vi "标样核查.vi"() -> ()   [LabVIEW 2016, in "斯坦道多参数.lvlib"]
panel:
  out "运行状态":u16(ring) items=["空闲", "水样测试", "标样核查"]
  out "seconds since 1Jan1904":timestamp
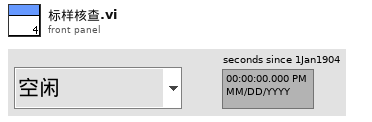
[diagram p1: front panel]
types:
  T1 = cluster{"ph":bool, "DO":bool, "Cond":bool, "Turb":bool, "叶绿素a":bool, "藻密度":bool, "ORP":bool, "cod":bool, "DO2":bool, "氯化物":bool, "氨氮":bool, "水中油":bool, "悬浮物":bool, "余氯":bool}
  T2 = cluster{"运行模式":enum16{"维护模式", "常规模式", "应急模式", "质控模式"}, "24H周期设置":bool[]}
  T3 = typedef "集成多参数单参数字段定义.ctl" = cluster{"时间":timestamp, "测量模式":string, "数据类型":string, "检测值":sgl, "单位":string, "数据标识":string, "信号值":sgl, "标样参考值":sgl, "因子编码":string, "探头温度":sgl, "LastTime":timestamp}
  T4 = cluster{"数据保存间隔":dbl, "保存组数":dbl, "水温标样值":dbl, "pH标样值":dbl, "溶解氧标样值":dbl, "电导率标样值":dbl, "浊度标样值":dbl, "悬浮物标样值":dbl, "叶绿素a标样值":dbl, "藻密度标样值":dbl, "ORP标样值":dbl, "氯化物标样值":dbl, "COD标样值":dbl, "氨氮标样值":dbl, "水中油标样值":dbl, "余氯标样值":dbl, "pH启用":bool, "溶解氧启用":bool, "电导率启用":bool, "浊度启用":bool, "悬浮物启用":bool, "叶绿素a启用":bool, "藻密度启用":bool, "ORP启用":bool, "氯化物启用":bool, "COD启用":bool, "氨氮启用":bool, "水中油启用":bool, "余氯启用":bool}
  T5 = typedef "LVDateTimeRec.ctl" = cluster{"秒数的小数部分":dbl, "秒":i32, "分":i32, "时":i32, "日":i32, "月":i32, "年":i32, "天数（周）":i32, "天数（年）":i32, "DST":i32}
  T6 = cluster{"温度测量值":sgl, "测量值":sgl, "温度偏移修正值":sgl, "信号值":sgl, "数据标识":string}
  T7 = cluster{"温度测量值":sgl, "DO%":sgl, "DOmg/L":sgl, "温度偏移修正值":sgl, "数据标识mg/L":string, "数据标识%":string}
  T8 = cluster{"CH":u16, "监测值":dbl, "信号值":sgl, "数据标识":string}
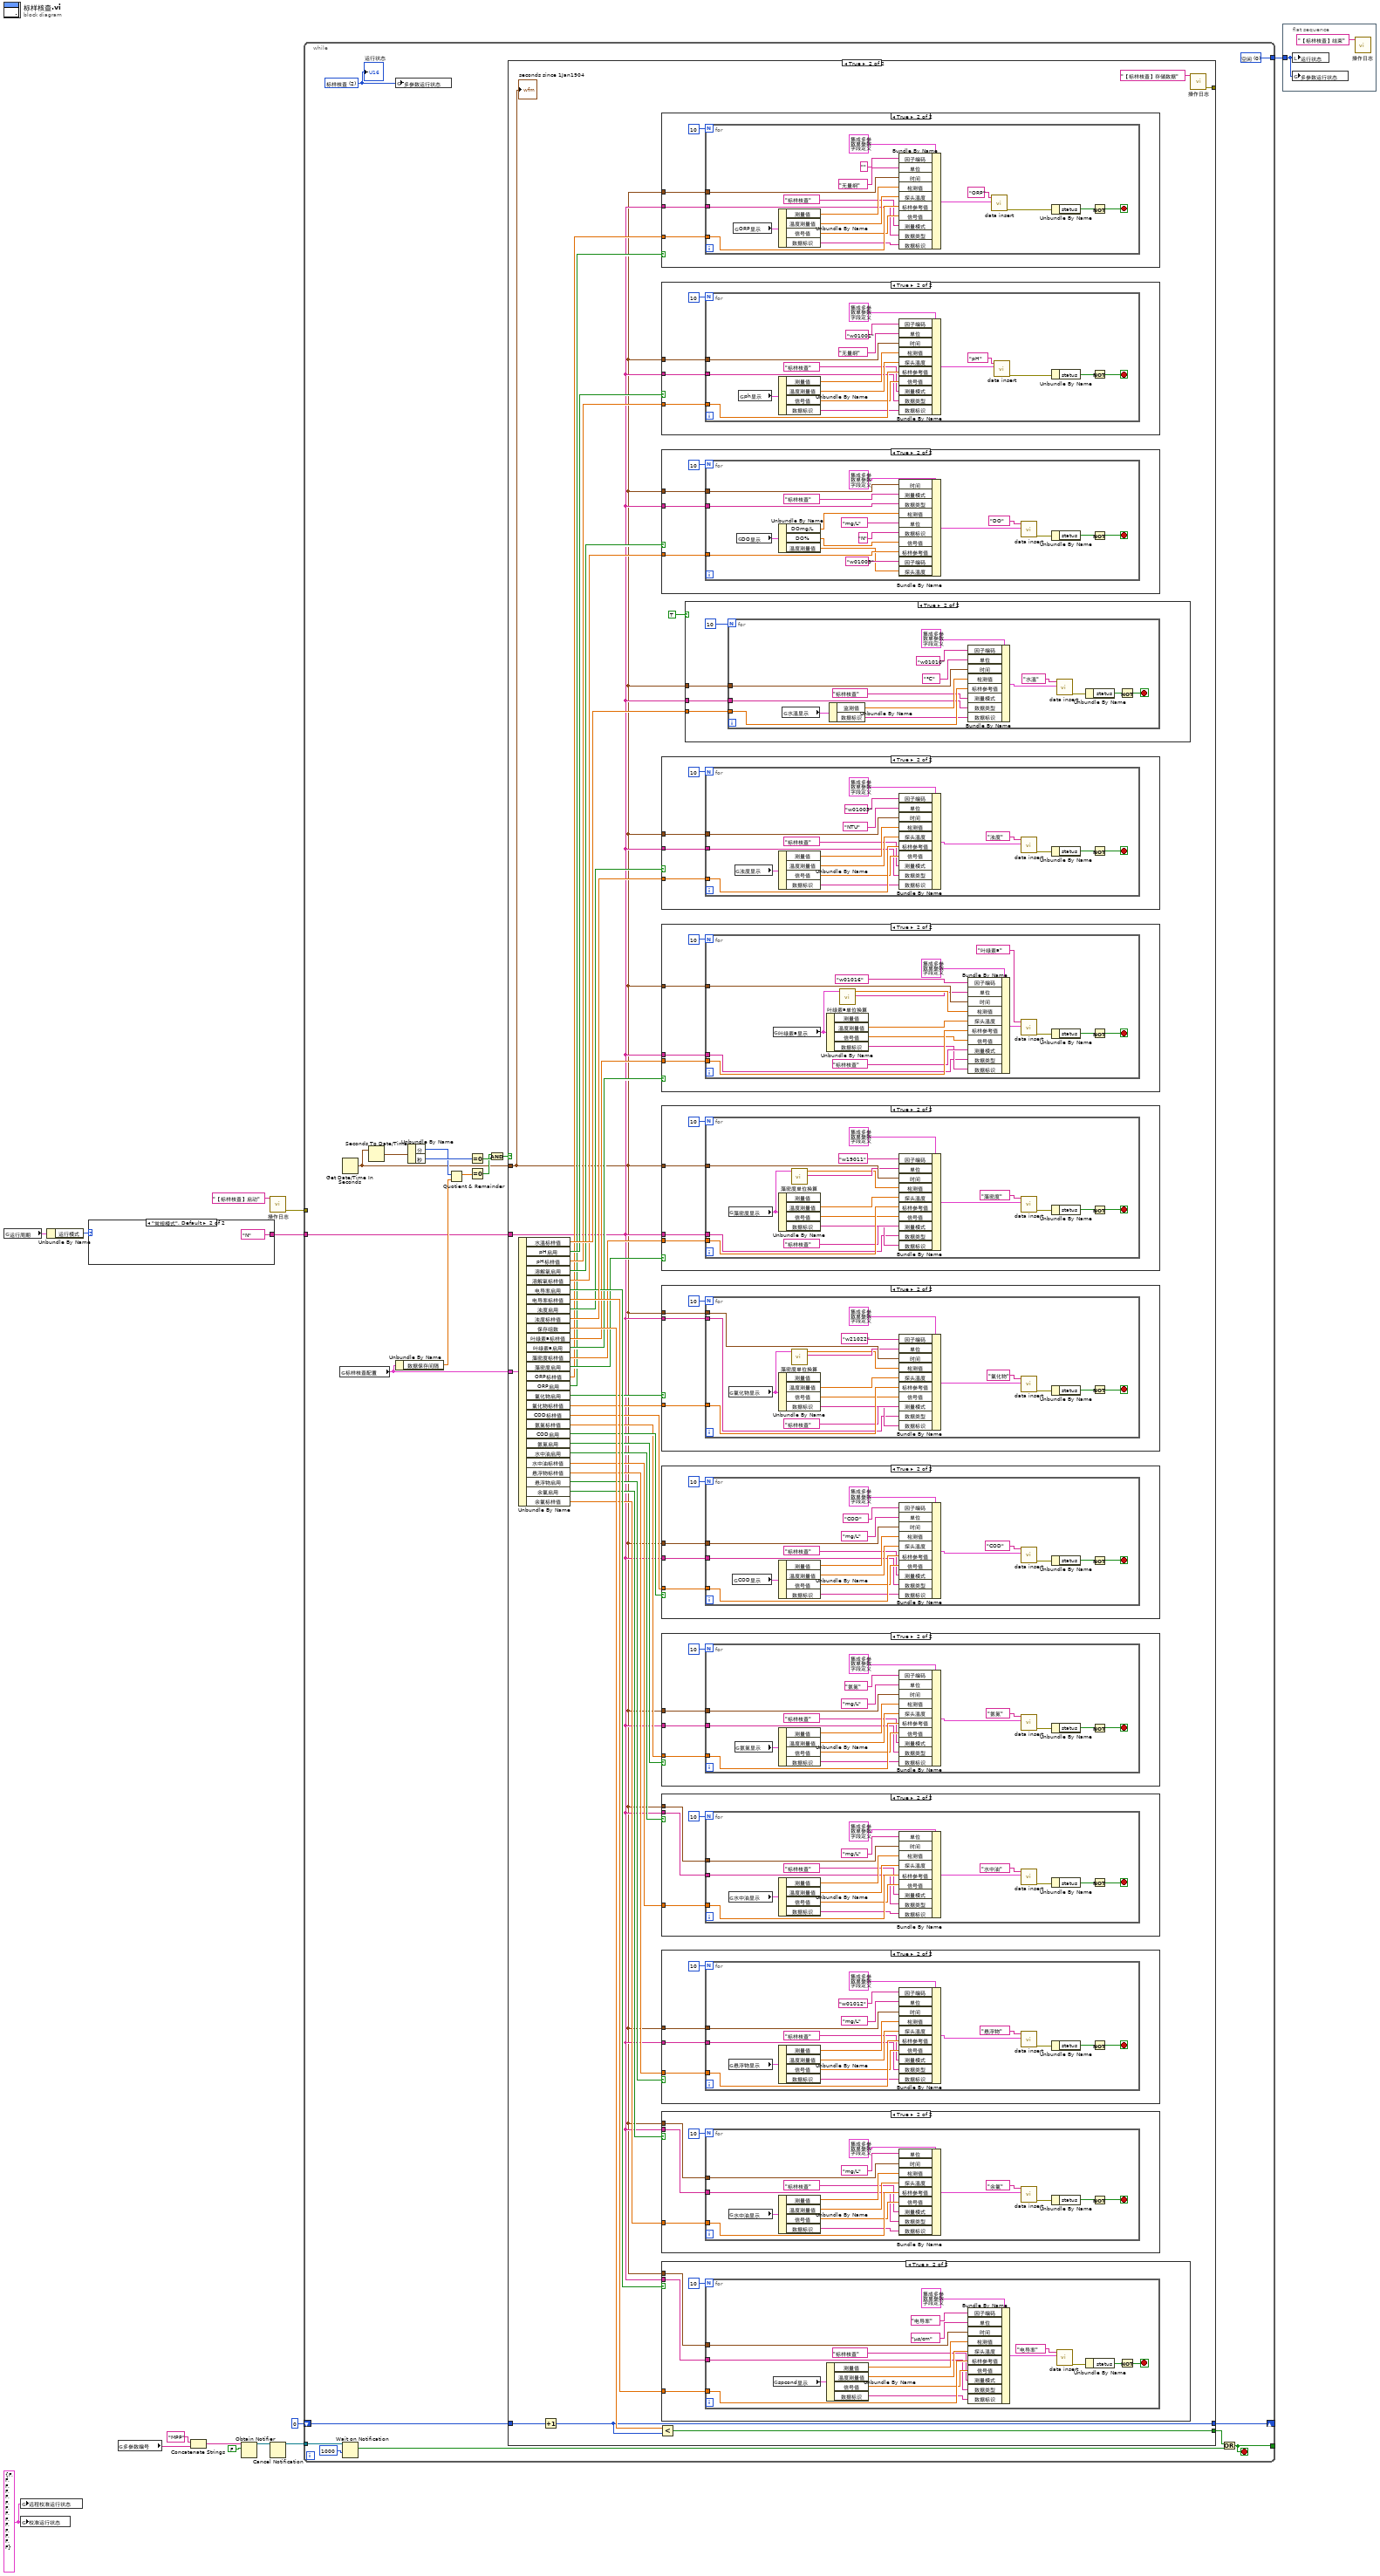
[diagram p0: block diagram]
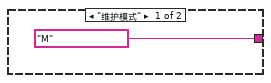
[diagram p2: hidden frame]
diagram:
  w1 = T1 {"ph"=FALSE, "DO"=FALSE, "Cond"=FALSE, "Turb"=FALSE, "叶绿素a"=FALSE, "藻密度"=FALSE, "ORP"=FALSE, "cod"=FALSE, "DO2"=FALSE, "氯化物"=FALSE, "氨氮"=FALSE, "水中油"=FALSE, "悬浮物"=FALSE, "余氯"=FALSE} ("远程校准运行状态")
  n1 = global read "断电保存变量.vi" "运行周期"() -> (w3:T2)
  n2 = global write "多参数全局变量.vi" "远程校准运行状态"(w1) -> ()
  n3 = global write "多参数全局变量.vi" "校准运行状态"(w1) -> ()
  n4 = Unbundle By Name(w3) -> ("运行模式"=w2:enum16{"维护模式", "常规模式", "应急模式", "质控模式"})
  n5 = case shown="\"常规模式\", Default" w2 {
    tunnel: ["M" ("数据标记表") "N" ("数据标记表")] -> w4
    frame "维护模式" {
    }
    frame "常规模式", Default {
    }
  }
  n6 = global read "多参数全局变量.vi" "多参数编号"() -> (w8:string)
  n7 = Concatenate Strings("MPP" ("名称（未命名）"), w8) -> (w9:string)
  n8 = Obtain Notifier(name (unnamed)=w9, notification data type=FALSE) -> (notifier out=w12:refnum<notifier>)  [unwired: 2 in, 2 out]
  n9 = call "操作日志.vi"("日志信息"="【标样核查】启动") -> ("error out"=w6:errorcluster)  [unwired: 10 in]
  n10 = Cancel Notification(0:w12) -> (8:w11:refnum<notifier>)  [unwired: 1 in, 2 out]
  n11 = while {
    tunnel: [w27] -> w10
    tunnel: w11 -> [w26]
    tunnel: w6 -> [_]
    shift-right: [w20] -> _
    shift-left: 0 -> [w21]
    tunnel: w4 -> [w18]
    tunnel: [w17] -> _
    stop <- w17 stop-if-true
    w27 = u16 0 items=["空闲", "水样测试", "标样核查"] ("多参数运行状态")
    w23 = u16 2 items=["空闲", "水样测试", "标样核查"] ("多参数运行状态")
    n12 = global read "断电保存变量.vi" "标样核查配置"() -> (w22:T4)
    n13 = Get Date/Time In Seconds() -> (seconds since 1Jan1904=w28:timestamp)
    n14 = Wait on Notification(notifier=w26, timeout in ms (-1)=1000 ("超时毫秒(-1)")) -> (notification=w24:bool)  [unwired: 2 in, 3 out]
    n15 = Seconds To Date/Time(time stamp (now)=w28) -> (date time rec=w36:T5)  [unwired: 1 in]
    n16 = global write "多参数全局变量.vi" "多参数运行状态"(w23) -> ()
    n17 = Unbundle By Name(w22) -> ("数据保存间隔"=w31:dbl)
    n18 = Unbundle By Name(w36) -> ("分"=w32:i32, "秒"=w35:i32)
    n19 = Quotient & Remainder(x=w32, y=w31) -> (x-y*floor(x/y)=w30:dbl)  [unwired: 1 out]
    n20 = Equal To 0?(x=w35) -> (x = 0?=w34:bool)
    n21 = Equal To 0?(x=w30) -> (x = 0?=w29:bool)
    n22 = And(x=w29, y=w34) -> (x .and. y?=w33:bool)
    n23 = case shown="True" w33 {
      tunnel: w22 -> [_ w74]
      tunnel: w28 -> [_ w38]
      tunnel: [_ w67] -> _
      tunnel: w21 -> [w37 w61]
      tunnel: [w37 w59] -> w20
      tunnel: [_ w58] -> w19
      tunnel: w18 -> [_ w39]
      frame False {
      }
      frame True {
        n24 = Unbundle By Name(w74) -> ("水温标样值"=w73:dbl, "pH启用"=w66:bool, "pH标样值"=w72:dbl, "溶解氧启用"=w64:bool, "溶解氧标样值"=w71:dbl, "电导率启用"=w63:bool, "电导率标样值"=w70:dbl, "浊度启用"=w62:bool, "浊度标样值"=w69:dbl, "保存组数"=w60:dbl, "叶绿素a标样值"=w57:dbl, "叶绿素a启用"=w54:bool, "藻密度标样值"=w56:dbl, "藻密度启用"=w55:bool, "ORP标样值"=w53:dbl, "ORP启用"=w52:bool, "氯化物启用"=w51:bool, "氯化物标样值"=w50:dbl, "COD标样值"=w48:dbl, "氨氮标样值"=w46:dbl, "COD启用"=w49:bool, "氨氮启用"=w47:bool, "水中油启用"=w44:bool, "水中油标样值"=w45:dbl, "悬浮物标样值"=w42:dbl, "悬浮物启用"=w43:bool, "余氯启用"=w41:bool, "余氯标样值"=w40:dbl)
        n25 = Increment(x=w61) -> (x+1=w59:i32)
        n26 = Less?(x=w60, y=w59) -> (x < y?=w58:bool)
        n27 = case shown="True" w52 {
          tunnel: w53 -> [_ w202]
          tunnel: w38 -> [_ w200]
          tunnel: w39 -> [_ w199]
          frame False {
          }
          frame True {
            n28 = for {
              N: 10 -> [_]
              tunnel: w202 -> [w218]
              tunnel: w200 -> [w211]
              tunnel: w199 -> [w206]
              stop <- w212 stop-if-true
              n29 = global read "多参数全局变量.vi" "ORP显示"() -> (w217:T6)
              n30 = Unbundle By Name(w217) -> ("测量值"=w216:sgl, "温度测量值"=w215:sgl, "信号值"=w209:sgl, "数据标识"=w207:string)
              n31 = Bundle By Name(cluster=T3 {"时间"=timestamp(0 s since 1904-01-01), "测量模式"="水样测试", "数据类型"="N", "检测值"=0.0, "单位"="mg/L", "数据标识"="N", "信号值"=0.0, "标样参考值"=0.0, "因子编码"="", "探头温度"=0.0, "LastTime"=timestamp(0 s since 1904-01-01)} ("data"), "因子编码"="", "单位"="无量纲", "时间"=w211, "检测值"=w216, "探头温度"=w215, "标样参考值"=w218, "信号值"=w209, "测量模式"="标样核查", "数据类型"=w206, "数据标识"=w207) -> (w210:T3)
              n32 = call "data insert.vi"("data"=w210, "table in"="ORP") -> ("error out"=w214:errorcluster)  [unwired: 9 in]
              n33 = Unbundle By Name(w214) -> ("status"=w213:bool)
              n34 = Not(x=w213) -> (.not. x?=w212:bool)
            }
          }
        }
        n35 = case shown="True" w66 {
          tunnel: w72 -> [_ w328]
          tunnel: w38 -> [_ w326]
          tunnel: w39 -> [_ w325]
          frame False {
          }
          frame True {
            n36 = for {
              N: 10 -> [_]
              tunnel: w328 -> [w342]
              tunnel: w326 -> [w335]
              tunnel: w325 -> [w330]
              stop <- w336 stop-if-true
              n37 = global read "多参数全局变量.vi" "ph显示"() -> (w341:T6)
              n38 = Unbundle By Name(w341) -> ("测量值"=w340:sgl, "温度测量值"=w339:sgl, "信号值"=w333:sgl, "数据标识"=w331:string)
              n39 = Bundle By Name(cluster=T3 {"时间"=timestamp(0 s since 1904-01-01), "测量模式"="水样测试", "数据类型"="N", "检测值"=0.0, "单位"="mg/L", "数据标识"="N", "信号值"=0.0, "标样参考值"=0.0, "因子编码"="", "探头温度"=0.0, "LastTime"=timestamp(0 s since 1904-01-01)} ("data"), "因子编码"="w01001", "单位"="无量纲", "时间"=w335, "检测值"=w340, "探头温度"=w339, "标样参考值"=w342, "信号值"=w333, "测量模式"="标样核查", "数据类型"=w330, "数据标识"=w331) -> (w334:T3)
              n40 = call "data insert.vi"("data"=w334, "table in"="pH" ("table输入")) -> ("error out"=w338:errorcluster)  [unwired: 9 in]
              n41 = Unbundle By Name(w338) -> ("status"=w337:bool)
              n42 = Not(x=w337) -> (.not. x?=w336:bool)
            }
          }
        }
        n43 = case shown="True" w64 {
          tunnel: w71 -> [_ w307]
          tunnel: w38 -> [_ w305]
          tunnel: w39 -> [_ w304]
          frame False {
          }
          frame True {
            n44 = for {
              N: 10 -> [_]
              tunnel: w307 -> [w314]
              tunnel: w305 -> [w319]
              tunnel: w304 -> [w309]
              stop <- w322 stop-if-true
              n45 = global read "多参数全局变量.vi" "DO显示"() -> (w324:T7)
              n46 = Unbundle By Name(w324) -> ("DOmg/L"=w317:sgl, "DO%"=w311:sgl, "温度测量值"=w310:sgl)
              n47 = Bundle By Name(cluster=T3 {"时间"=timestamp(0 s since 1904-01-01), "测量模式"="水样测试", "数据类型"="N", "检测值"=0.0, "单位"="mg/L", "数据标识"="N", "信号值"=0.0, "标样参考值"=0.0, "因子编码"="", "探头温度"=0.0, "LastTime"=timestamp(0 s since 1904-01-01)} ("data"), "时间"=w319, "测量模式"="标样核查", "数据类型"=w309, "检测值"=w317, "单位"="mg/L", "数据标识"="N" ("水样数据标识"), "信号值"=w311, "标样参考值"=w314, "因子编码"="w01009", "探头温度"=w310) -> (w320:T3)
              n48 = call "data insert.vi"("data"=w320, "table in"="DO") -> ("error out"=w312:errorcluster)  [unwired: 9 in]
              n49 = Unbundle By Name(w312) -> ("status"=w323:bool)
              n50 = Not(x=w323) -> (.not. x?=w322:bool)
            }
          }
        }
        n51 = case shown="True" w62 {
          tunnel: w69 -> [_ w265]
          tunnel: w38 -> [_ w263]
          tunnel: w39 -> [_ w262]
          frame False {
          }
          frame True {
            n52 = for {
              N: 10 -> [_]
              tunnel: w265 -> [w278]
              tunnel: w263 -> [w271]
              tunnel: w262 -> [w267]
              stop <- w272 stop-if-true
              n53 = global read "多参数全局变量.vi" "浊度显示"() -> (w277:T6)
              n54 = Unbundle By Name(w277) -> ("测量值"=w276:sgl, "温度测量值"=w275:sgl, "信号值"=w270:sgl, "数据标识"=w268:string)
              n55 = Bundle By Name(cluster=T3 {"时间"=timestamp(0 s since 1904-01-01), "测量模式"="水样测试", "数据类型"="N", "检测值"=0.0, "单位"="mg/L", "数据标识"="N", "信号值"=0.0, "标样参考值"=0.0, "因子编码"="", "探头温度"=0.0, "LastTime"=timestamp(0 s since 1904-01-01)} ("data"), "因子编码"="w01003", "单位"="NTU", "时间"=w271, "检测值"=w276, "探头温度"=w275, "标样参考值"=w278, "信号值"=w270, "测量模式"="标样核查", "数据类型"=w267, "数据标识"=w268) -> (w281:T3)
              n56 = call "data insert.vi"("data"=w281, "table in"="浊度" ("table输入")) -> ("error out"=w274:errorcluster)  [unwired: 9 in]
              n57 = Unbundle By Name(w274) -> ("status"=w273:bool)
              n58 = Not(x=w273) -> (.not. x?=w272:bool)
            }
          }
        }
        n59 = case shown="True" w54 {
          tunnel: w57 -> [_ w244]
          tunnel: w38 -> [_ w242]
          tunnel: w39 -> [_ w241]
          frame False {
          }
          frame True {
            n60 = for {
              N: 10 -> [_]
              tunnel: w244 -> [w258]
              tunnel: w242 -> [w253]
              tunnel: w241 -> [w249]
              stop <- w254 stop-if-true
              n61 = global read "多参数全局变量.vi" "叶绿素a显示"() -> (w247:T6)
              n62 = Unbundle By Name(w247) -> ("温度测量值"=w257:sgl, "信号值"=w252:sgl, "数据标识"=w250:string)  [unwired: 1 out]
              n63 = call "叶绿素a单位换算.vi"("叶绿素a显示"=w247) -> ("检测值1.单位"=w245:string, "测量值"=w246:sgl)  [unwired: 8 in, 1 out]
              n64 = Bundle By Name(cluster=T3 {"时间"=timestamp(0 s since 1904-01-01), "测量模式"="水样测试", "数据类型"="N", "检测值"=0.0, "单位"="mg/L", "数据标识"="N", "信号值"=0.0, "标样参考值"=0.0, "因子编码"="", "探头温度"=0.0, "LastTime"=timestamp(0 s since 1904-01-01)} ("data"), "因子编码"="w01016", "单位"=w245, "时间"=w253, "检测值"=w246, "探头温度"=w257, "标样参考值"=w258, "信号值"=w252, "测量模式"="标样核查", "数据类型"=w249, "数据标识"=w250) -> (w261:T3)
              n65 = call "data insert.vi"("data"=w261, "table in"="叶绿素a" ("table输入")) -> ("error out"=w256:errorcluster)  [unwired: 9 in]
              n66 = Unbundle By Name(w256) -> ("status"=w255:bool)
              n67 = Not(x=w255) -> (.not. x?=w254:bool)
            }
          }
        }
        n68 = case shown="True" w55 {
          tunnel: w56 -> [_ w223]
          tunnel: w38 -> [_ w221]
          tunnel: w39 -> [_ w220]
          frame False {
          }
          frame True {
            n69 = for {
              N: 10 -> [_]
              tunnel: w223 -> [w237]
              tunnel: w221 -> [w232]
              tunnel: w220 -> [w228]
              stop <- w233 stop-if-true
              n70 = global read "多参数全局变量.vi" "藻密度显示"() -> (w226:T6)
              n71 = Unbundle By Name(w226) -> ("温度测量值"=w236:sgl, "信号值"=w231:sgl, "数据标识"=w229:string)  [unwired: 1 out]
              n72 = call "藻密度单位换算.vi"("藻密度显示"=w226) -> ("检测值1.单位"=w225:string, "测量值"=w224:sgl)  [unwired: 8 in, 1 out]
              n73 = Bundle By Name(cluster=T3 {"时间"=timestamp(0 s since 1904-01-01), "测量模式"="水样测试", "数据类型"="N", "检测值"=0.0, "单位"="mg/L", "数据标识"="N", "信号值"=0.0, "标样参考值"=0.0, "因子编码"="", "探头温度"=0.0, "LastTime"=timestamp(0 s since 1904-01-01)} ("data"), "因子编码"="w19011", "单位"=w225, "时间"=w232, "检测值"=w224, "探头温度"=w236, "标样参考值"=w237, "信号值"=w231, "测量模式"="标样核查", "数据类型"=w228, "数据标识"=w229) -> (w240:T3)
              n74 = call "data insert.vi"("data"=w240, "table in"="藻密度" ("table输入")) -> ("error out"=w235:errorcluster)  [unwired: 9 in]
              n75 = Unbundle By Name(w235) -> ("status"=w234:bool)
              n76 = Not(x=w234) -> (.not. x?=w233:bool)
            }
          }
        }
        n77 = case shown="True" w51 {
          tunnel: w50 -> [_ w181]
          tunnel: w38 -> [_ w179]
          tunnel: w39 -> [_ w178]
          frame False {
          }
          frame True {
            n78 = for {
              N: 10 -> [_]
              tunnel: w181 -> [w197]
              tunnel: w179 -> [w192]
              tunnel: w178 -> [w188]
              stop <- w193 stop-if-true
              n79 = global read "多参数全局变量.vi" "氯化物显示"() -> (w186:T6)
              n80 = Unbundle By Name(w186) -> ("温度测量值"=w196:sgl, "信号值"=w191:sgl, "数据标识"=w189:string)  [unwired: 1 out]
              n81 = call "藻密度单位换算.vi"("藻密度显示"=w186) -> ("检测值1.单位"=w185:string, "测量值"=w184:sgl)  [unwired: 8 in, 1 out]
              n82 = Bundle By Name(cluster=T3 {"时间"=timestamp(0 s since 1904-01-01), "测量模式"="水样测试", "数据类型"="N", "检测值"=0.0, "单位"="mg/L", "数据标识"="N", "信号值"=0.0, "标样参考值"=0.0, "因子编码"="", "探头温度"=0.0, "LastTime"=timestamp(0 s since 1904-01-01)} ("data"), "因子编码"="w21022", "单位"=w185, "时间"=w192, "检测值"=w184, "探头温度"=w196, "标样参考值"=w197, "信号值"=w191, "测量模式"="标样核查", "数据类型"=w188, "数据标识"=w189) -> (w198:T3)
              n83 = call "data insert.vi"("data"=w198, "table in"="氯化物") -> ("error out"=w195:errorcluster)  [unwired: 9 in]
              n84 = Unbundle By Name(w195) -> ("status"=w194:bool)
              n85 = Not(x=w194) -> (.not. x?=w193:bool)
            }
          }
        }
        n86 = case shown="True" w49 {
          tunnel: w48 -> [_ w160]
          tunnel: w38 -> [_ w158]
          tunnel: w39 -> [_ w157]
          frame False {
          }
          frame True {
            n87 = for {
              N: 10 -> [_]
              tunnel: w160 -> [w174]
              tunnel: w158 -> [w167]
              tunnel: w157 -> [w162]
              stop <- w168 stop-if-true
              n88 = global read "多参数全局变量.vi" "COD显示"() -> (w173:T6)
              n89 = Unbundle By Name(w173) -> ("测量值"=w172:sgl, "温度测量值"=w171:sgl, "信号值"=w165:sgl, "数据标识"=w163:string)
              n90 = Bundle By Name(cluster=T3 {"时间"=timestamp(0 s since 1904-01-01), "测量模式"="水样测试", "数据类型"="N", "检测值"=0.0, "单位"="mg/L", "数据标识"="N", "信号值"=0.0, "标样参考值"=0.0, "因子编码"="", "探头温度"=0.0, "LastTime"=timestamp(0 s since 1904-01-01)} ("data"), "因子编码"="COD", "单位"="mg/L", "时间"=w167, "检测值"=w172, "探头温度"=w171, "标样参考值"=w174, "信号值"=w165, "测量模式"="标样核查", "数据类型"=w162, "数据标识"=w163) -> (w177:T3)
              n91 = call "data insert.vi"("data"=w177, "table in"="COD" ("table输入")) -> ("error out"=w170:errorcluster)  [unwired: 9 in]
              n92 = Unbundle By Name(w170) -> ("status"=w169:bool)
              n93 = Not(x=w169) -> (.not. x?=w168:bool)
            }
          }
        }
        n94 = case shown="True" w47 {
          tunnel: w46 -> [_ w139]
          tunnel: w38 -> [_ w137]
          tunnel: w39 -> [_ w136]
          frame False {
          }
          frame True {
            n95 = for {
              N: 10 -> [_]
              tunnel: w139 -> [w153]
              tunnel: w137 -> [w146]
              tunnel: w136 -> [w141]
              stop <- w147 stop-if-true
              n96 = global read "多参数全局变量.vi" "氨氮显示"() -> (w152:T6)
              n97 = Unbundle By Name(w152) -> ("测量值"=w151:sgl, "温度测量值"=w150:sgl, "信号值"=w144:sgl, "数据标识"=w142:string)
              n98 = Bundle By Name(cluster=T3 {"时间"=timestamp(0 s since 1904-01-01), "测量模式"="水样测试", "数据类型"="N", "检测值"=0.0, "单位"="mg/L", "数据标识"="N", "信号值"=0.0, "标样参考值"=0.0, "因子编码"="", "探头温度"=0.0, "LastTime"=timestamp(0 s since 1904-01-01)} ("data"), "因子编码"="氨氮", "单位"="mg/L", "时间"=w146, "检测值"=w151, "探头温度"=w150, "标样参考值"=w153, "信号值"=w144, "测量模式"="标样核查", "数据类型"=w141, "数据标识"=w142) -> (w156:T3)
              n99 = call "data insert.vi"("data"=w156, "table in"="氨氮" ("table输入")) -> ("error out"=w149:errorcluster)  [unwired: 9 in]
              n100 = Unbundle By Name(w149) -> ("status"=w148:bool)
              n101 = Not(x=w148) -> (.not. x?=w147:bool)
            }
          }
        }
        n102 = case shown="True" w44 {
          tunnel: w45 -> [_ w119]
          tunnel: w38 -> [_ w117]
          tunnel: w39 -> [_ w116]
          frame False {
          }
          frame True {
            n103 = for {
              N: 10 -> [_]
              tunnel: w119 -> [w133]
              tunnel: w117 -> [w126]
              tunnel: w116 -> [w121]
              stop <- w127 stop-if-true
              n104 = global read "多参数全局变量.vi" "水中油显示"() -> (w132:T6)
              n105 = Unbundle By Name(w132) -> ("测量值"=w131:sgl, "温度测量值"=w130:sgl, "信号值"=w124:sgl, "数据标识"=w122:string)
              n106 = Bundle By Name(cluster=T3 {"时间"=timestamp(0 s since 1904-01-01), "测量模式"="水样测试", "数据类型"="N", "检测值"=0.0, "单位"="mg/L", "数据标识"="N", "信号值"=0.0, "标样参考值"=0.0, "因子编码"="", "探头温度"=0.0, "LastTime"=timestamp(0 s since 1904-01-01)} ("data"), "单位"="mg/L", "时间"=w126, "检测值"=w131, "探头温度"=w130, "标样参考值"=w133, "信号值"=w124, "测量模式"="标样核查", "数据类型"=w121, "数据标识"=w122) -> (w135:T3)
              n107 = call "data insert.vi"("data"=w135, "table in"="水中油" ("table输入")) -> ("error out"=w129:errorcluster)  [unwired: 9 in]
              n108 = Unbundle By Name(w129) -> ("status"=w128:bool)
              n109 = Not(x=w128) -> (.not. x?=w127:bool)
            }
          }
        }
        n110 = case shown="True" w43 {
          tunnel: w42 -> [_ w98]
          tunnel: w38 -> [_ w96]
          tunnel: w39 -> [_ w95]
          frame False {
          }
          frame True {
            n111 = for {
              N: 10 -> [_]
              tunnel: w98 -> [w112]
              tunnel: w96 -> [w105]
              tunnel: w95 -> [w100]
              stop <- w106 stop-if-true
              n112 = global read "多参数全局变量.vi" "悬浮物显示"() -> (w111:T6)
              n113 = Unbundle By Name(w111) -> ("测量值"=w110:sgl, "温度测量值"=w109:sgl, "信号值"=w103:sgl, "数据标识"=w101:string)
              n114 = Bundle By Name(cluster=T3 {"时间"=timestamp(0 s since 1904-01-01), "测量模式"="水样测试", "数据类型"="N", "检测值"=0.0, "单位"="mg/L", "数据标识"="N", "信号值"=0.0, "标样参考值"=0.0, "因子编码"="", "探头温度"=0.0, "LastTime"=timestamp(0 s since 1904-01-01)} ("data"), "因子编码"="w01012", "单位"="mg/L", "时间"=w105, "检测值"=w110, "探头温度"=w109, "标样参考值"=w112, "信号值"=w103, "测量模式"="标样核查", "数据类型"=w100, "数据标识"=w101) -> (w115:T3)
              n115 = call "data insert.vi"("data"=w115, "table in"="悬浮物" ("table输入")) -> ("error out"=w108:errorcluster)  [unwired: 9 in]
              n116 = Unbundle By Name(w108) -> ("status"=w107:bool)
              n117 = Not(x=w107) -> (.not. x?=w106:bool)
            }
          }
        }
        n118 = case shown="True" w41 {
          tunnel: w40 -> [_ w78]
          tunnel: w38 -> [_ w76]
          tunnel: w39 -> [_ w75]
          frame False {
          }
          frame True {
            n119 = for {
              N: 10 -> [_]
              tunnel: w78 -> [w92]
              tunnel: w76 -> [w85]
              tunnel: w75 -> [w80]
              stop <- w86 stop-if-true
              n120 = global read "多参数全局变量.vi" "水中油显示"() -> (w91:T6)
              n121 = Unbundle By Name(w91) -> ("测量值"=w90:sgl, "温度测量值"=w89:sgl, "信号值"=w83:sgl, "数据标识"=w81:string)
              n122 = Bundle By Name(cluster=T3 {"时间"=timestamp(0 s since 1904-01-01), "测量模式"="水样测试", "数据类型"="N", "检测值"=0.0, "单位"="mg/L", "数据标识"="N", "信号值"=0.0, "标样参考值"=0.0, "因子编码"="", "探头温度"=0.0, "LastTime"=timestamp(0 s since 1904-01-01)} ("data"), "单位"="mg/L", "时间"=w85, "检测值"=w90, "探头温度"=w89, "标样参考值"=w92, "信号值"=w83, "测量模式"="标样核查", "数据类型"=w80, "数据标识"=w81) -> (w94:T3)
              n123 = call "data insert.vi"("data"=w94, "table in"="余氯" ("table输入")) -> ("error out"=w88:errorcluster)  [unwired: 9 in]
              n124 = Unbundle By Name(w88) -> ("status"=w87:bool)
              n125 = Not(x=w87) -> (.not. x?=w86:bool)
            }
          }
        }
        n126 = case shown="True" w63 {
          tunnel: w70 -> [_ w286]
          tunnel: w38 -> [_ w284]
          tunnel: w39 -> [_ w283]
          frame False {
          }
          frame True {
            n127 = for {
              N: 10 -> [_]
              tunnel: w286 -> [w300]
              tunnel: w284 -> [w293]
              tunnel: w283 -> [w288]
              stop <- w294 stop-if-true
              n128 = global read "多参数全局变量.vi" "spcond显示"() -> (w299:T6)
              n129 = Unbundle By Name(w299) -> ("测量值"=w298:sgl, "温度测量值"=w297:sgl, "信号值"=w291:sgl, "数据标识"=w289:string)
              n130 = Bundle By Name(cluster=T3 {"时间"=timestamp(0 s since 1904-01-01), "测量模式"="水样测试", "数据类型"="N", "检测值"=0.0, "单位"="mg/L", "数据标识"="N", "信号值"=0.0, "标样参考值"=0.0, "因子编码"="", "探头温度"=0.0, "LastTime"=timestamp(0 s since 1904-01-01)} ("data"), "因子编码"="电导率", "单位"="μs/cm", "时间"=w293, "检测值"=w298, "探头温度"=w297, "标样参考值"=w300, "信号值"=w291, "测量模式"="标样核查", "数据类型"=w288, "数据标识"=w289) -> (w303:T3)
              n131 = call "data insert.vi"("data"=w303, "table in"="电导率" ("table输入")) -> ("error out"=w296:errorcluster)  [unwired: 9 in]
              n132 = Unbundle By Name(w296) -> ("status"=w295:bool)
              n133 = Not(x=w295) -> (.not. x?=w294:bool)
            }
          }
        }
        n134 = case shown="True" TRUE {
          tunnel: w73 -> [_ w349]
          tunnel: w38 -> [_ w348]
          tunnel: w39 -> [_ w346]
          frame False {
          }
          frame True {
            n135 = for {
              N: 10 -> [_]
              tunnel: w349 -> [w360]
              tunnel: w348 -> [w357]
              tunnel: w346 -> [w351]
              stop <- w354 stop-if-true
              n136 = global read "多参数全局变量.vi" "水温显示"() -> (w359:T8)
              n137 = Unbundle By Name(w359) -> ("监测值"=w358:dbl, "数据标识"=w352:string)
              n138 = Bundle By Name(cluster=T3 {"时间"=timestamp(0 s since 1904-01-01), "测量模式"="水样测试", "数据类型"="N", "检测值"=0.0, "单位"="mg/L", "数据标识"="N", "信号值"=0.0, "标样参考值"=0.0, "因子编码"="", "探头温度"=0.0, "LastTime"=timestamp(0 s since 1904-01-01)} ("data"), "因子编码"="w01010", "单位"="℃", "时间"=w357, "检测值"=w358, "标样参考值"=w360, "测量模式"="标样核查", "数据类型"=w351, "数据标识"=w352) -> (w363:T3)
              n139 = call "data insert.vi"("data"=w363, "table in"="水温" ("table输入")) -> ("error out"=w356:errorcluster)  [unwired: 9 in]
              n140 = Unbundle By Name(w356) -> ("status"=w355:bool)
              n141 = Not(x=w355) -> (.not. x?=w354:bool)
            }
          }
        }
        n142 = call "操作日志.vi"("日志信息"="【标样核查】存储数据") -> ("error out"=w67:errorcluster)  [unwired: 10 in]
        "seconds since 1Jan1904" <- w38
      }
    }
    n143 = Or(x=w19, y=w24) -> (x .or. y?=w17:bool)
    "运行状态" <- w23
  }
  n144 = flat-sequence {
    tunnel: w10 -> [w366]
    frame #0 {
      n145 = local write "运行状态"(w366) -> ()
      n146 = global write "多参数全局变量.vi" "多参数运行状态"(w366) -> ()
      n147 = call "操作日志.vi"("日志信息"="【标样核查】结束") -> ()  [unwired: 10 in, 1 out]
    }
  }
